vi "Get Diameter from Voltage.vi"(8 "error in":errorcluster, 10 "Vin":dbl, 11 "DMA in":refnum<class "DMA.lvclass">) -> (0 "error out":errorcluster, 2 "Dout":dbl, 3 "DMA out":refnum<class "DMA.lvclass">)   [LabVIEW 2015, in "DMA.lvclass"]
doc: "Retrieve the calculated diameter from a given voltage. This is done by setting the theoretical electrical mobility calculated from the voltage to the particle mobility (Zv = Zd). The diameter returned will also be a function of the ambient flow properties. This includes temperature, pressure and flow rates."
uses:
  DMA.lvclass
  DMA.lvclass/DMA.ctl
  Dz from V.vi
  <vilib>/gmath/zero.llb/Newton Raphson Zero Finder (VI).vi
  <vilib>/gmath/NI_Gmath.lvlib
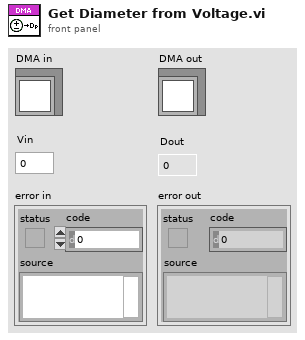
[diagram p1: front panel]
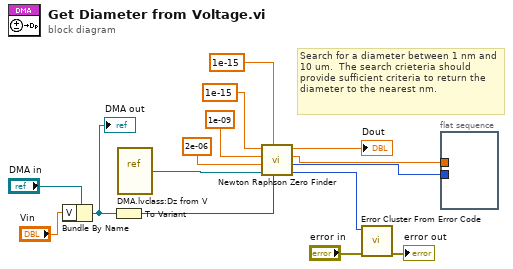
[diagram p0: block diagram]
diagram:
  # "Search for a diameter between 1 nm and 10 um.  The search crieteria should provide sufficient criteria to return the diameter to the nearest nm."
  n1 = Bundle By Name(cluster="DMA in", "V"="Vin") -> (w5:refnum<class "DMA.lvclass">)
  "DMA out" <- w5
  n2 = To Variant(anything=w5) -> (Variant=w13:variant)
  n3 = vi-ref "DMA.lvclass:Dz from V.vi"() -> (w4:refnum<vi>)
  n4 = call-poly <vilib>:"Newton Raphson Zero Finder.vi"("data"=w13, "accuracy"=1e-15, "f(x)"=w4, "end"=2e-06, "start"=1e-09, "h"=1e-15) -> ("error"=w8:i32, "ticks"=w1:u32, "f(zero)"=w2:dbl, "zero"=→"Dout":dbl)  [unwired: 2 in]
  n5 = call <vilib>:"Error Cluster From Error Code.vi"("error in (no error)"="error in", "error code (0)"=w8) -> ("error out"=→"error out":errorcluster)  [unwired: 7 in]
  n6 = flat-sequence {
    tunnel: w2 -> [_]
    tunnel: w1 -> [_]
    frame #0 {
    }
  }
